vi "Emballage check code lu_FLATPROP.vi"(1 "tab pcs emballées historique":string[][](array[string])=[["112105740008090004", "01.01.2001 01:01:00", "55", "01234/08-01.01.01", "1", "0"], ["112105740008090006", "01.01.2001 01:01:00", "55", "56789/08-01.01.01", "3", "0"], ["112105740008090007", "01.01.2001 01:01:00", "55", "56789/08-01.01.01", "4", "0"], ["112105740008090007", "01.01.2001 01:01:00", "55", "00123/08-01.01.01", "2", "1"]], 2 "error in":errorcluster caption="entrée d'erreur", 3 "n° lot à scanner":string="0808", 4 "chaîne lue par le lecteur IN":string="112105740008090004", 5 "tab pcs déjà emballées (histo+actu)":string[](array[string])=["112105740008090009", "112105740008090004", "112105740008090006", "112105740008090007", "112105740008090007R1"], 6 "Quantité du lot de livraison":string="200", 11 "Pb réseau GPAO":bool, 16 "n° commande EC":string="R03838/08-01.01.01") -> (9 "error out":errorcluster caption="sortie d'erreur", 13 "offset sur code bar début index":i16=-1, 14 "largeur index":i16=-1, 15 "Date production de la piéce":string, 17 "chaîne lue par le lecteur OUT":string="112105740008090004R1", 18 "Arrêter la série (T)":bool, 19 "Paramètres OK(=> T)":bool)   [LabVIEW 2020]
uses:
  Instance           3 31Saved   Emballage check code lu .vi
  VG_VerifTests_ModeRetour.vi
  Modules/FS/60_FS_Controles/60_FS_SetGet.ctl
panel:
  out "Glissière 2":u8(slide)=100 caption="Identification terminé." scale=0.0..100.0
  out "RETOUR CLIENT":string="1"
  # "dans historique :\ncolonne 0 = numéro de pièce\ncolonne 1 = date\ncolonne 2 = visa emball\ncolonne 3 = No commande\ncolonne 4 = carton\ncolonne 5 = qtté cmdée ou RC"
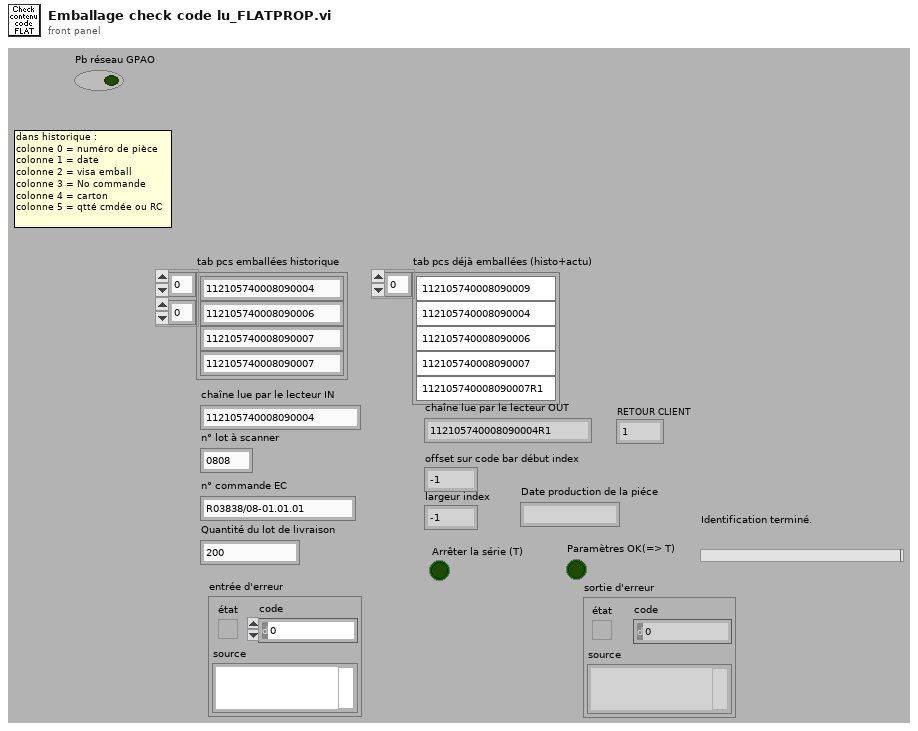
[diagram p1: front panel]
types:
  T1 = typedef "60_FS_SetGet.ctl" = enum16{"set", "get"}
  T2 = typedef "60_FS_CLT_Chemins.ctl" = cluster{"Racine_local":path, "Racine_reseau":path, "Racine_Support_Application":path, "Fichier_Journalisation":path, "Connexion_BDD_VSX":path, "Connexion_BDD_PLZ":path}
  T3 = typedef "Emballage_BDD_param_Produit.ctl" = cluster{"No_Valve_FAS":string, "suffixe":string, "designation":string, "indice_produit":string, "code_barre_fixe":string, "affiche_code_barre_client":string, "affiche_no_client":string, "Nb_vlve_par_carton":u16, "melange_des_lots_possible":string, "id_article":string, "Indice_Rev":string, "Famille":string, "date":string, "code_barre_fixe_Fin":string, "Longeur_No_Serie":string}
  T4 = typedef "DATA Valve.ctl" = cluster{"Existe ?":bool, "N° Valve":string, "Valve Codif":string, "Résultat test Hyst.":i32, "Résultat test Fuite":i32, "ID Valid Flatprop M":i32, "Date test Hyst.":string, "Date Test Fuite":string, "Date Emballage":string, "Historique Test Hyst.":string, "Historique Tes Fuite":string, "N° RETOUR":string, "Résultat test Dielec.":i32, "Date Test Dielec.":string, "R Test Dielec.[Ohm]":dbl, "Ifuite Test Dielec. [mA]":dbl, "Q Test Dielec.[L/mn]":dbl, "N°Valve sans Embase":string}
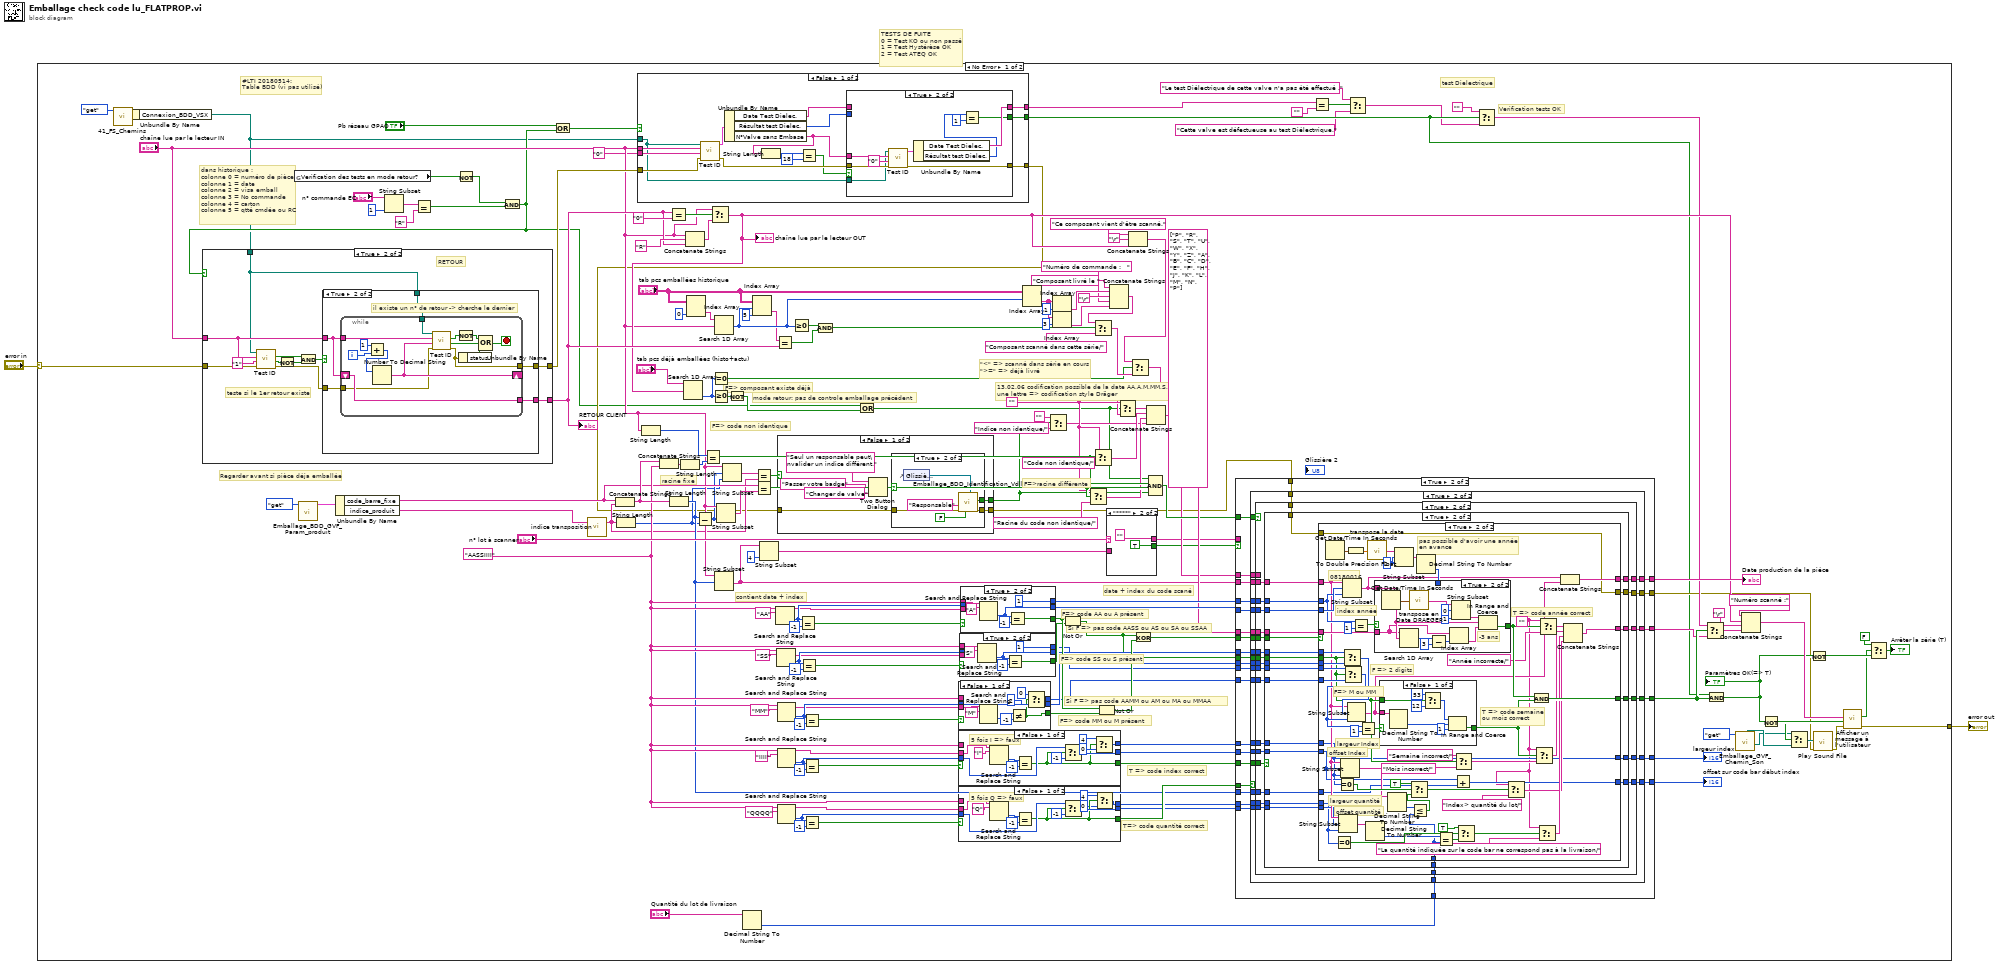
[diagram p0: block diagram]
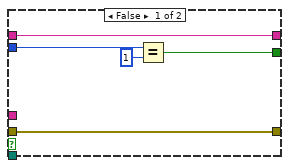
[diagram p2: hidden frame]
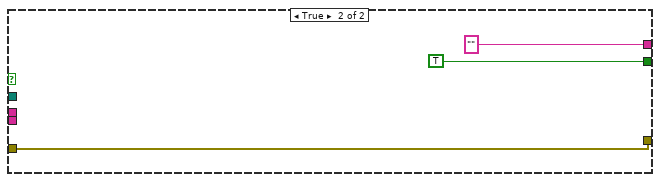
[diagram p3: hidden frame]
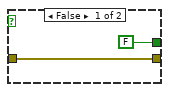
[diagram p4: hidden frame]
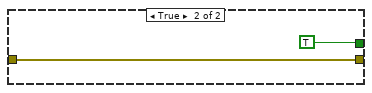
[diagram p5: hidden frame]
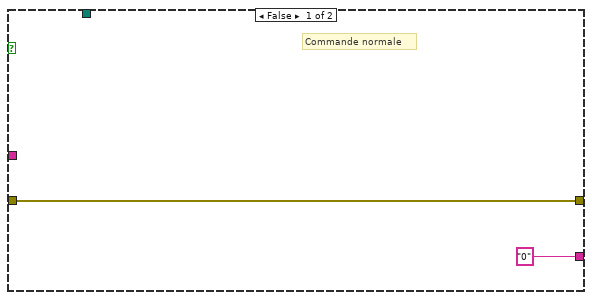
[diagram p6: hidden frame]
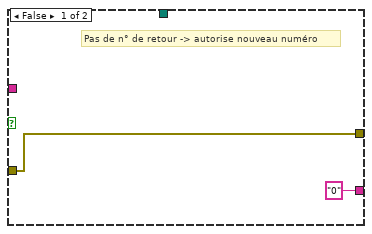
[diagram p7: hidden frame]
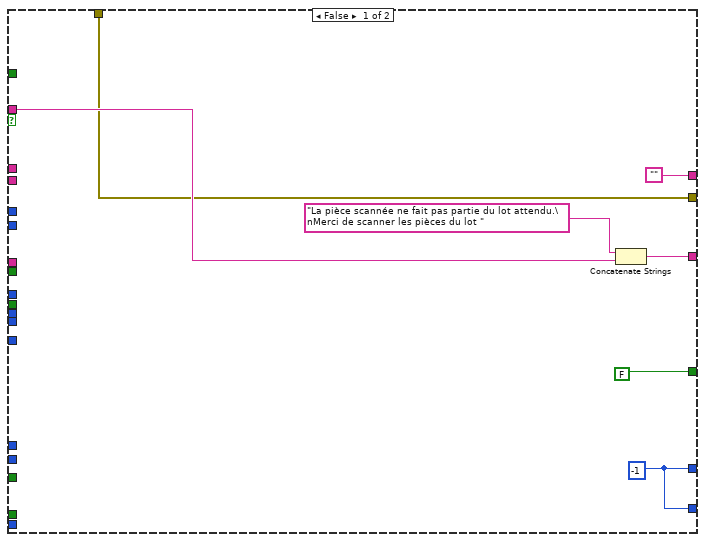
[diagram p8: hidden frame]
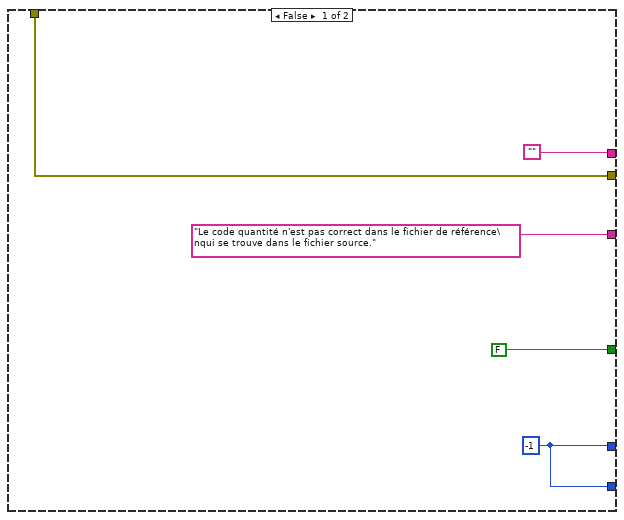
[diagram p9: hidden frame]
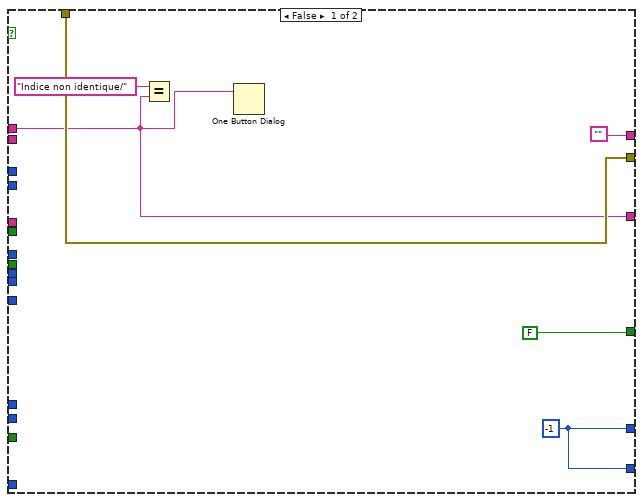
[diagram p10: hidden frame]
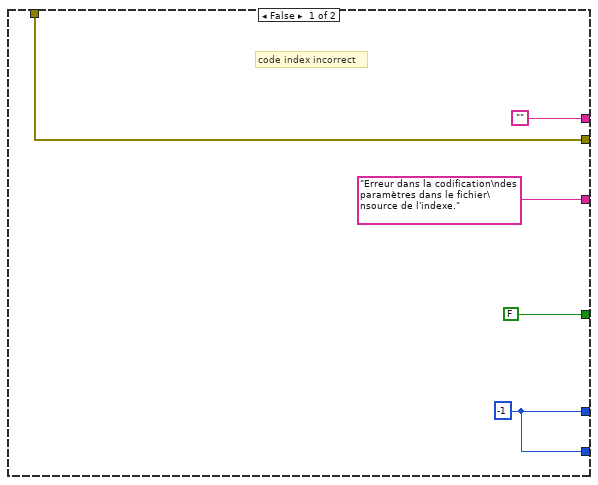
[diagram p11: hidden frame]
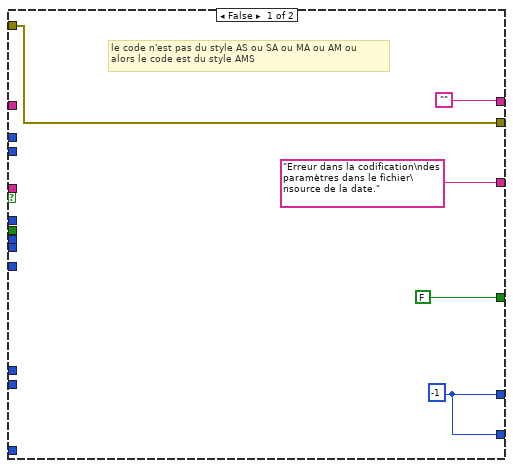
[diagram p12: hidden frame]
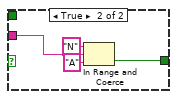
[diagram p13: hidden frame]
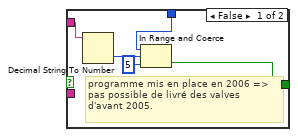
[diagram p14: hidden frame]
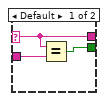
[diagram p15: hidden frame]
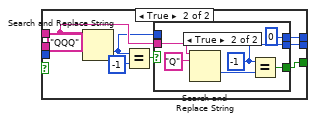
[diagram p16: hidden frame]
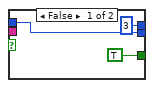
[diagram p17: hidden frame]
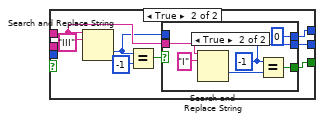
[diagram p18: hidden frame]
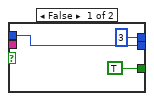
[diagram p19: hidden frame]
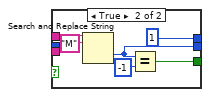
[diagram p20: hidden frame]
diagram:
  # "TESTS DE FUITE\n0 = Test KO ou non passé\n1 = Test Hystérèse OK\n2 = Test ATEQ OK"
  n1 = case shown="No Error" "error in" {
    selector: "error in" -> [w12 w577]
    tunnel: [w50 w577] -> w1
    frame No Error {
      w52 = "AASSIIII"
      w131 = ""
      # "#LTI 20180514:\nTable BDD (vi pas utilisé)"
      # "mode retour: pas de controle emballage précédent"
      # "Regarder avant si pièce déja emballée"
      # "Verification tests OK"
      # "test Dielectrique"
      # "dans historique :\ncolonne 0 = numéro de pièce\ncolonne 1 = date\ncolonne 2 = visa emball\ncolonne 3 = No commande\ncolonne 4 = carton\ncolonne 5 = qtté cmdée ou RC"
      # "\"<\" => scanné dans série en cours\n\">=\" => déjà livré"
      # "T=> code quantité correct"
      # "Si F => pas code AASS ou AS ou SA ou SSAA"
      # "Si F => pas code AAMM ou AM ou MA ou MMAA"
      # "F=> code MM ou M présent"
      # "F=> code SS ou S présent"
      # "F=> code AA ou A présent"
      # "T => code index correct"
      # "13.02.06 codification possible de la date AA,A,M,MM,S,SS\nune lettre => codification style Dräger"
      # "date + index du code scané"
      # "contient date + index"
      # "racine fixe"
      # "F=> composant existe déjà"
      # "F=> code non identique"
      # "F=>racine différente"
      n2 = call "41_FS_Chemins.vi"("SetGet"=60_FS_SetGet."get") -> ("CLT_Chemins_out"=w6:T2)  [unwired: 9 in, 1 out]
      n3 = Unbundle By Name(w6) -> ("Connexion_BDD_VSX"=w5:path)
      n4 = global read "VG_VerifTests_ModeRetour.vi" "Verification des tests en mode retour?"() -> (w14:bool)
      n5 = call "Emballage_BDD_GVF_Param_produit.vi"("Énum"=enum16{"set", "get"}."get") -> ("CLS_param_produit"=w3:T3)  [unwired: 7 in, 3 out]
      n6 = Unbundle By Name(w3) -> ("code_barre_fixe"=w42:string, "indice_produit"=w41:string)
      n7 = String Subset(string="n° commande EC", length (rest)=1 ("longueur (reste)")) -> (substring=w65:string)  [unwired: 1 in]
      n8 = Equal?(x=w65, y="R" ("expression régulière")) -> (x = y?=w23:bool)
      n9 = Not(x=w14) -> (.not. x?=w13:bool)
      n10 = And(x=w13, y=w23) -> (x .and. y?=w11:bool)
      n11 = case shown="True" w11 {
        tunnel: "chaîne lue par le lecteur IN" -> [_ w231]
        tunnel: ["0" ("expression régulière") w227] -> w54
        tunnel: w5 -> [_ w226]
        tunnel: w12 -> [w221 w225]
        tunnel: [w221 w223] -> w49
        frame False {
          # "Commande normale"
        }
        frame True {
          # "teste si le 1er retour existe"
          # "RETOUR"
          n12 = call "Test ID.vi"("error in"=w225, "NO_RETOUR"="1" ("expression régulière"), "NO_VALVE"=w231, "connection information"=w226) -> ("error out"=w224:errorcluster, "Erreur de\n comunication"=w229:bool, "Existe ?"=w233:bool)  [unwired: 1 out]
          n13 = Not(x=w229) -> (.not. x?=w228:bool)
          n14 = And(x=w233, y=w228) -> (x .and. y?=w232:bool)
          n15 = case shown="True" w232 {
            tunnel: w226 -> [_ w240]
            tunnel: w231 -> [_ w239]
            tunnel: ["0" ("expression régulière") w238] -> w227
            tunnel: w224 -> [w234 w237]
            tunnel: [w234 w236] -> w223
            frame False {
              # "Pas de n° de retour -> autorise nouveau numéro"
            }
            frame True {
              # "il existe un n° de retour -> cherche le dernier"
              n16 = while {
                tunnel: w239 -> [w247]
                shift-right: [w249] -> _
                shift-left: w239 -> [w248]
                tunnel: w240 -> [w251]
                tunnel: [w248] -> w238
                tunnel: w237 -> [w243]
                tunnel: [w242] -> w236
                i -> [w254]
                stop <- w246 stop-if-true
                n17 = Add(x=1, y=w254) -> (x+y=w252:i32)
                n18 = Number To Decimal String(number=w252) -> (decimal integer string=w249:string)  [unwired: 1 in]
                n19 = call "Test ID.vi"("error in"=w243, "NO_RETOUR"=w249, "NO_VALVE"=w247, "connection information"=w251) -> ("error out"=w242:errorcluster, "Erreur de\n comunication"=w253:bool, "Existe ?"=w245:bool)  [unwired: 1 out]
                n20 = Not(x=w245) -> (.not. x?=w244:bool)
                n21 = Unbundle By Name(w242) -> ("status"=w241:bool)
                n22 = Compound Arithmetic op=OR(w244, w253, w241) -> (w246:bool)
              }
            }
          }
        }
      }
      "RETOUR CLIENT" <- w54
      n23 = Or(x="Pb réseau GPAO", y=w11) -> (x .or. y?=w26:bool)
      n24 = call "indice transposition.vi"("indice entrée"=w41) -> ("indice corrigé"=w36:string)  [unwired: 1 in, 1 out]
      n25 = Concatenate Strings(w42, w36) -> (w80:string)
      n26 = String Length(string=w36) -> (length=w38:i32)
      n27 = case shown="False" w26 {
        tunnel: "chaîne lue par le lecteur IN" -> [w184 _]
        tunnel: "0" ("chaîne lue par le lecteur IN") -> [w183 _]
        tunnel: w5 -> [w175 _]
        tunnel: w49 -> [w182 w203]
        tunnel: [w180 w203] -> w29
        tunnel: [w173 "" ("Date Test Dielec.")] -> w22
        tunnel: [w172 TRUE] -> w19
        frame False {
          n28 = call "Test ID.vi"("error in"=w182, "NO_RETOUR"=w183, "NO_VALVE"=w184, "connection information"=w175) -> ("error out"=w181:errorcluster, "TEST ID VALID"=w185:T4)  [unwired: 2 out]
          n29 = Unbundle By Name(w185) -> ("Date Test Dielec."=w174:string, "Résultat test Dielec."=w171:i32, "N°Valve sans Embase"=w177:string)
          n30 = String Length(string=w177) -> (length=w179:i32)
          n31 = Equal?(x=w179, y=18) -> (x = y?=w176:bool)
          n32 = case shown="True" w176 {
            tunnel: w181 -> [w190 w199]
            tunnel: [w190 w198] -> w180
            tunnel: w177 -> [_ w196]
            tunnel: w175 -> [_ w195]
            tunnel: [w189 w194] -> w173
            tunnel: w174 -> [w189 _]
            tunnel: [w187 w191] -> w172
            tunnel: w171 -> [w186 _]
            frame False {
              n33 = Equal?(x=w186, y=1) -> (x = y?=w187:bool)
            }
            frame True {
              n34 = call "Test ID.vi"("error in"=w199, "NO_RETOUR"="0", "NO_VALVE"=w196, "connection information"=w195) -> ("error out"=w198:errorcluster, "TEST ID VALID"=w197:T4)  [unwired: 2 out]
              n35 = Unbundle By Name(w197) -> ("Date Test Dielec."=w194:string, "Résultat test Dielec."=w192:i32)
              n36 = Equal?(x=w192, y=1) -> (x = y?=w191:bool)
            }
          }
        }
        frame True {
        }
      }
      n37 = String Length(string="chaîne lue par le lecteur IN") -> (length=w169:i32)
      n38 = Concatenate Strings(w80, w52) -> (w170:string)
      n39 = Equal?(x=w54, y="0" ("chaîne")) -> (x = y?=w55:bool)
      n40 = String Length(string=w80) -> (length=w43:i32)
      n41 = String Length(string=w170) -> (length=w168:i32)
      n42 = Concatenate Strings("chaîne lue par le lecteur IN", "R" ("chaîne"), w54) -> (w53:string)
      n43 = Index Array(array="tab pcs emballées historique", index (col)=0) -> (element=w88:string[])  [unwired: 1 in]
      n44 = Subtract(x=w43, y=w38) -> (x-y=w39:i32)
      n45 = Equal?(x=w169, y=w168) -> (x = y?=w136:bool)
      n46 = Select(t="chaîne lue par le lecteur IN", s=w55, f=w53) -> (s? t:f=w51:string)
      "chaîne lue par le lecteur OUT" <- w51
      n47 = Search 1D Array(1D array="tab pcs déjà emballées (histo+actu)", element=w51) -> (index of element=w87:i32)  [unwired: 1 in]
      n48 = Equal To 0?(x=w87) -> (x = 0?=w84:bool)
      n49 = Greater Or Equal To 0?(x=w87) -> (x >= 0?=w135:bool)
      n50 = Search 1D Array(1D array=w88, element="chaîne lue par le lecteur IN") -> (index of element=w63:i32)  [unwired: 1 in]
      n51 = String Subset(string="chaîne lue par le lecteur IN", offset (0)=w43) -> (substring=w77:string)  [unwired: 1 in]
      n52 = String Subset(string="chaîne lue par le lecteur IN", length (rest)=w39) -> (substring=w167:string)  [unwired: 1 in]
      n53 = String Subset(string="chaîne lue par le lecteur IN", offset (0)=w39, length (rest)=w38) -> (substring=w37:string)
      n54 = Not(x=w135) -> (.not. x?=w134:bool)
      n55 = Decimal String To Number(string="Quantité du lot de livraison") -> (number=w122:i32)  [unwired: 2 in, 1 out]
      n56 = Index Array(array="tab pcs emballées historique", index (row)=w63, index (col)=5) -> (element=w61:string)
      n57 = Equal?(x=w42, y=w167) -> (x = y?=w137:bool)
      n58 = Equal?(x=w37, y=w36) -> (x = y?=w30:bool)
      n59 = String Subset(string=w77, length (rest)=4 ("longueur (reste)")) -> (substring=w72:string)  [unwired: 1 in]
      n60 = Equal?(x=w61, y=w54) -> (x = y?=w60:bool)
      n61 = Search and Replace String(input string=w52, search string="AA") -> (result string=w125:string, offset past replacement=w154:i32)  [unwired: 6 in, 2 out]
      n62 = Search and Replace String(input string=w52, search string="SS") -> (result string=w110:string, offset past replacement=w153:i32)  [unwired: 6 in, 2 out]
      n63 = case shown="False" w30 {
        tunnel: w29 -> [w210 w220]
        tunnel: [w209 w220] -> w28
        tunnel: [w208 TRUE] -> w27
        frame False {
          n64 = Two Button Dialog(message="Seul un responsable peut\nvalider un indice différent.", 1:"Changer de valve" ("Nom du bouton F (\"Annuler\")"), 2:"Passer votre badge" ("Nom du bouton V (\"OK\")")) -> (T button?=w207:bool)
          n65 = case shown="True" w207 {
            tunnel: w210 -> [w212 w215]
            tunnel: [w212 w214] -> w209
            tunnel: [FALSE ("OK") w213] -> w208
            frame False {
            }
            frame True {
              n66 = control-ref of="Glissière 2"() -> (w218:refnum<vi>)
              n67 = call "Emballage_BDD_Identification_Vdll.vi"("Glissière"=w218, "lecture seul possible ?"=FALSE, "error in"=w215, "Posage choisi"="Responsable" ("Posage choissi")) -> ("error Out"=w214:errorcluster, "OK"=w213:bool)  [unwired: 3 in, 3 out]
            }
          }
        }
        frame True {
        }
      }
      n68 = Search and Replace String(input string=w52, search string="MM") -> (result string=w109:string, offset past replacement=w152:i32)  [unwired: 6 in, 2 out]
      n69 = Search and Replace String(input string=w52, search string="IIII") -> (result string=w126:string, offset past replacement=w119:i32)  [unwired: 6 in, 2 out]
      n70 = Search and Replace String(input string=w52, search string="QQQQ") -> (result string=w117:string, offset past replacement=w116:i32)  [unwired: 6 in, 2 out]
      n71 = Greater Or Equal To 0?(x=w63) -> (x >= 0?=w59:bool)
      n72 = Equal?(x=w154, y=-1) -> (x = y?=w159:bool)
      n73 = Equal?(x=w153, y=-1) -> (x = y?=w160:bool)
      n74 = Equal?(x=w152, y=-1) -> (x = y?=w158:bool)
      n75 = Equal?(x=w119, y=-1) -> (x = y?=w155:bool)
      n76 = Equal?(x=w116, y=-1) -> (x = y?=w111:bool)
      n77 = And(x=w59, y=w60) -> (x .and. y?=w58:bool)
      n78 = Or(x=w11, y=w134) -> (x .or. y?=w24:bool)
      n79 = case shown="False" w155 {
        tunnel: w52 -> [_ w519]
        tunnel: [w505 w518] -> w120
        tunnel: w126 -> [w511 _]
        tunnel: w119 -> [w510 _]
        tunnel: [w508 w516] -> w118
        tunnel: [w504 w515] -> w113
        frame False {
          # "5 fois I => faux"
          n80 = Search and Replace String(input string=w511, search string="I") -> (offset past replacement=w512:i32)  [unwired: 6 in, 3 out]
          n81 = Equal?(x=w512, y=-1) -> (x = y?=w505:bool)
          n82 = Select(t=w510, s=w505, f=-1) -> (s? t:f=w508:i32)
          n83 = Select(t=4, s=w505, f=0) -> (s? t:f=w504:i32)
        }
        frame True {
          n84 = Search and Replace String(input string=w519, search string="III") -> (offset past replacement=w517:i32)  [unwired: 6 in, 3 out]
          n85 = Equal?(x=w517, y=-1) -> (x = y?=w520:bool)
          n86 = case shown="True" w520 {
            tunnel: w519 -> [_ w530]
            tunnel: [TRUE w528] -> w518
            tunnel: w517 -> [w524 _]
            tunnel: [w524 w527] -> w516
            tunnel: [3 0] -> w515
            frame False {
            }
            frame True {
              w527 = -1
              n87 = Search and Replace String(input string=w530, search string="I") -> (offset past replacement=w529:i32)  [unwired: 6 in, 3 out]
              n88 = Equal?(x=w527, y=w529) -> (x = y?=w528:bool)
            }
          }
        }
      }
      n89 = case shown="False" w111 {
        tunnel: w52 -> [_ w491]
        tunnel: [w479 w490] -> w115
        tunnel: w117 -> [w483 _]
        tunnel: w116 -> [w482 _]
        tunnel: [w480 w488] -> w114
        tunnel: [w476 w487] -> w112
        frame False {
          # "5 fois Q => faux"
          n90 = Search and Replace String(input string=w483, search string="Q") -> (offset past replacement=w484:i32)  [unwired: 6 in, 3 out]
          n91 = Equal?(x=w484, y=-1) -> (x = y?=w479:bool)
          n92 = Select(t=w482, s=w479, f=-1) -> (s? t:f=w480:i32)
          n93 = Select(t=4, s=w479, f=0) -> (s? t:f=w476:i32)
        }
        frame True {
          n94 = Search and Replace String(input string=w491, search string="QQQ") -> (offset past replacement=w489:i32)  [unwired: 6 in, 3 out]
          n95 = Equal?(x=w489, y=-1) -> (x = y?=w492:bool)
          n96 = case shown="True" w492 {
            tunnel: w491 -> [_ w502]
            tunnel: [TRUE w500] -> w490
            tunnel: w489 -> [w496 _]
            tunnel: [w496 w499] -> w488
            tunnel: [3 0] -> w487
            frame False {
            }
            frame True {
              w499 = -1
              n97 = Search and Replace String(input string=w502, search string="Q") -> (offset past replacement=w501:i32)  [unwired: 6 in, 3 out]
              n98 = Equal?(x=w499, y=w501) -> (x = y?=w500:bool)
            }
          }
        }
      }
      n99 = case shown="False" w158 {
        tunnel: w52 -> [_ w546]
        tunnel: [w533 w543] -> w151
        tunnel: [w540 w542] -> w143
        tunnel: w152 -> [w540 _]
        tunnel: [w535 1] -> w140
        tunnel: w109 -> [w536 _]
        frame False {
          n100 = Search and Replace String(input string=w536, search string="M") -> (offset past replacement=w539:i32)  [unwired: 6 in, 3 out]
          n101 = Not Equal?(x=w539, y=-1) -> (x != y?=w533:bool)
          n102 = Select(t=0, s=w533, f=2) -> (s? t:f=w535:i32)
        }
        frame True {
          n103 = Search and Replace String(input string=w546, search string="M") -> (offset past replacement=w542:i32)  [unwired: 6 in, 3 out]
          n104 = Equal?(x=w542, y=-1) -> (x = y?=w543:bool)
        }
      }
      n105 = case shown="True" w160 {
        tunnel: w52 -> [_ w561]
        tunnel: w153 -> [w555 _]
        tunnel: [w555 w558] -> w144
        tunnel: [w547 w557] -> w149
        tunnel: [w550 1] -> w141
        tunnel: w110 -> [w551 _]
        frame False {
          n106 = Search and Replace String(input string=w551, search string="S") -> (offset past replacement=w552:i32)  [unwired: 6 in, 3 out]
          n107 = Not Equal?(x=w552, y=-1) -> (x != y?=w547:bool)
          n108 = Select(t=0, s=w547, f=2) -> (s? t:f=w550:i32)
        }
        frame True {
          n109 = Search and Replace String(input string=w561, search string="S") -> (offset past replacement=w558:i32)  [unwired: 6 in, 3 out]
          n110 = Equal?(x=w558, y=-1) -> (x = y?=w557:bool)
        }
      }
      n111 = case shown="True" w159 {
        tunnel: w52 -> [_ w575]
        tunnel: w154 -> [w570 _]
        tunnel: [w570 w573] -> w146
        tunnel: [w562 w572] -> w150
        tunnel: [w565 1] -> w145
        tunnel: w125 -> [w568 _]
        frame False {
          n112 = Search and Replace String(input string=w568, search string="A") -> (offset past replacement=w566:i32)  [unwired: 6 in, 3 out]
          n113 = Not Equal?(x=w566, y=-1) -> (x != y?=w562:bool)
          n114 = Select(t=0, s=w562, f=2) -> (s? t:f=w565:i32)
        }
        frame True {
          n115 = Search and Replace String(input string=w575, search string="A") -> (offset past replacement=w573:i32)  [unwired: 6 in, 3 out]
          n116 = Equal?(x=w573, y=-1) -> (x = y?=w572:bool)
        }
      }
      n117 = Index Array(array="tab pcs emballées historique", index (row)=w63) -> (element=w90:string[])  [unwired: 1 in]
      n118 = Select(t="", s=w27, f="Indice non identique/") -> (s? t:f=w33:string)
      n119 = Index Array(array=w90, index=1) -> (element=w93:string)
      n120 = Index Array(array=w90, index=3) -> (element=w71:string)
      n121 = Not Or(1:w149, 2:w150) -> (0:w142:bool)
      n122 = Select(t=w131, s=w137, f="Racine du code non identique/") -> (s? t:f=w128:string)
      n123 = Select(t=w131, s=w136, f="Code non identique/") -> (s? t:f=w129:string)
      n124 = Not Or(1:w151, 2:w150) -> (0:w148:bool)
      n125 = case shown="\"****\"" "n° lot à scanner" {
        selector: "n° lot à scanner" -> [w471 _]
        tunnel: [w473 TRUE] -> w75
        tunnel: [w471 "" ("n° lot à scanner")] -> w74
        tunnel: w72 -> [w472 _]
        frame Default {
          n126 = Equal?(x=w471, y=w472) -> (x = y?=w473:bool)
        }
        frame "****" {
        }
      }
      n127 = Concatenate Strings("Composant livré le ", w93, "\r", "Numéro de commande :   ", w71) -> (w92:string)
      n128 = Select(t=w92, s=w58, f="Composant scanné dans cette série/") -> (s? t:f=w85:string)
      n129 = Concatenate Strings("Ce composant vient d'être scanné.", "\r", w51) -> (w82:string)
      n130 = Select(t=w82, s=w84, f=w85) -> (s? t:f=w86:string)
      n131 = Select(t=w131, s=w24, f=w86) -> (s? t:f=w130:string)
      n132 = Exclusive Or(1:w148, 2:w142) -> (0:w147:bool)
      n133 = Concatenate Strings(w130, w129, w128, w33) -> (w127:string)
      n134 = Compound Arithmetic op=AND(w24, w136, w137, w27) -> (w138:bool)
      n135 = case shown="True" w75 {
        tunnel: w147 -> [_ w288]
        tunnel: w146 -> [_ w287]
        tunnel: w145 -> [_ w286]
        tunnel: w144 -> [_ w285]
        tunnel: w143 -> [_ w284]
        tunnel: w142 -> [_ w283]
        tunnel: w141 -> [_ w282]
        tunnel: w140 -> [_ w281]
        tunnel: string[] ["P", "R", "S", "T", "U", "W", "X", "Y", "Z", "A", "B", "C", "D", "E", "F", "H", "J", "K", "L", "M", "N", "P"] -> [_ w280]
        tunnel: w138 -> [_ w279]
        tunnel: w127 -> [_ w278]
        tunnel: w122 -> [_ w277]
        tunnel: w120 -> [_ w276]
        tunnel: w118 -> [_ w275]
        tunnel: w115 -> [_ w274]
        tunnel: w114 -> [_ w273]
        tunnel: w113 -> [_ w272]
        tunnel: w112 -> [_ w271]
        tunnel: w43 -> [_ w270]
        tunnel: [w259 w269] -> w108
        tunnel: [w259 w268] -> w107
        tunnel: [w258 w267] -> w46
        tunnel: ["" w266] -> w98
        tunnel: [FALSE w265] -> w47
        tunnel: w77 -> [_ w264]
        tunnel: w74 -> [w256 _]
        tunnel: w28 -> [w255 w263]
        tunnel: [w255 w262] -> w32
        frame False {
          w259 = -1
          n136 = Concatenate Strings("La pièce scannée ne fait pas partie du lot attendu.\nMerci de scanner les pièces du lot ", w256) -> (w258:string)
        }
        frame True {
          n137 = case shown="True" w274 {
            tunnel: w276 -> [_ w319]
            tunnel: w288 -> [_ w318]
            tunnel: w287 -> [_ w317]
            tunnel: w286 -> [_ w316]
            tunnel: w285 -> [_ w315]
            tunnel: w284 -> [_ w314]
            tunnel: w283 -> [_ w313]
            tunnel: w282 -> [_ w312]
            tunnel: w281 -> [_ w311]
            tunnel: w264 -> [_ w310]
            tunnel: w280 -> [_ w309]
            tunnel: w279 -> [_ w308]
            tunnel: w278 -> [_ w307]
            tunnel: ["Le code quantité n'est pas correct dans le fichier de référence\nqui se trouve dans le fichier source." w306] -> w267
            tunnel: [FALSE w305] -> w265
            tunnel: w277 -> [_ w304]
            tunnel: w275 -> [_ w303]
            tunnel: w273 -> [_ w302]
            tunnel: w272 -> [_ w301]
            tunnel: w271 -> [_ w300]
            tunnel: ["" w299] -> w266
            tunnel: w270 -> [_ w298]
            tunnel: [w290 w297] -> w269
            tunnel: [w290 w296] -> w268
            tunnel: w263 -> [w289 w295]
            tunnel: [w289 w294] -> w262
            frame False {
              w290 = -1
            }
            frame True {
              n138 = case shown="True" w308 {
                tunnel: w319 -> [_ w349]
                tunnel: w318 -> [_ w348]
                tunnel: w317 -> [_ w347]
                tunnel: w316 -> [_ w346]
                tunnel: w315 -> [_ w345]
                tunnel: w314 -> [_ w344]
                tunnel: w313 -> [_ w343]
                tunnel: w312 -> [_ w342]
                tunnel: w311 -> [_ w341]
                tunnel: w310 -> [_ w340]
                tunnel: w309 -> [_ w339]
                tunnel: w307 -> [w320 _]
                tunnel: [w320 w337] -> w306
                tunnel: [FALSE w338] -> w305
                tunnel: w304 -> [_ w336]
                tunnel: w303 -> [_ w335]
                tunnel: w302 -> [_ w334]
                tunnel: w301 -> [_ w333]
                tunnel: w300 -> [_ w332]
                tunnel: ["" w331] -> w299
                tunnel: w298 -> [_ w330]
                tunnel: [w324 w329] -> w297
                tunnel: [w324 w328] -> w296
                tunnel: w295 -> [w322 w327]
                tunnel: [w322 w326] -> w294
                frame False {
                  w324 = -1
                  n139 = Equal?(x="Indice non identique/", y=w320) -> ()  [unwired: 1 out]
                  n140 = One Button Dialog(message=w320) -> ()  [unwired: 1 in, 1 out]
                }
                frame True {
                  n141 = case shown="True" w349 {
                    tunnel: w348 -> [_ w377]
                    tunnel: w347 -> [_ w376]
                    tunnel: w346 -> [_ w375]
                    tunnel: w345 -> [_ w374]
                    tunnel: w344 -> [_ w373]
                    tunnel: w343 -> [_ w372]
                    tunnel: w342 -> [_ w371]
                    tunnel: w341 -> [_ w370]
                    tunnel: w340 -> [_ w369]
                    tunnel: w339 -> [_ w368]
                    tunnel: [FALSE w367] -> w338
                    tunnel: ["Erreur dans la codification\ndes paramètres dans le fichier\nsource de l'indexe." w366] -> w337
                    tunnel: w336 -> [_ w365]
                    tunnel: w335 -> [_ w364]
                    tunnel: w334 -> [_ w363]
                    tunnel: w333 -> [_ w362]
                    tunnel: w332 -> [_ w361]
                    tunnel: ["" w360] -> w331
                    tunnel: w330 -> [_ w359]
                    tunnel: [w351 w358] -> w329
                    tunnel: [w351 w357] -> w328
                    tunnel: w327 -> [w350 w356]
                    tunnel: [w350 w355] -> w326
                    frame False {
                      w351 = -1
                      # "code index incorrect"
                    }
                    frame True {
                      n142 = case shown="True" w377 {
                        tunnel: w376 -> [_ w437]
                        tunnel: w375 -> [_ w429]
                        tunnel: w374 -> [_ w441]
                        tunnel: w373 -> [_ w440]
                        tunnel: w372 -> [_ w413]
                        tunnel: w371 -> [_ w439]
                        tunnel: w370 -> [_ w438]
                        tunnel: w369 -> [_ w409]
                        tunnel: w368 -> [_ w427]
                        tunnel: [FALSE w421] -> w367
                        tunnel: ["Erreur dans la codification\ndes paramètres dans le fichier\nsource de la date." w417] -> w366
                        tunnel: w365 -> [_ w396]
                        tunnel: w364 -> [_ w388]
                        tunnel: w363 -> [_ w408]
                        tunnel: w362 -> [_ w385]
                        tunnel: w361 -> [_ w407]
                        tunnel: ["" w389] -> w360
                        tunnel: w359 -> [_ w387]
                        tunnel: [w379 w386] -> w358
                        tunnel: [w379 w385] -> w357
                        tunnel: w356 -> [w378 w384]
                        tunnel: [w378 w384] -> w355
                        frame False {
                          w379 = -1
                          # "le code n'est pas du style AS ou SA ou MA ou AM ou\nalors le code est du style AMS"
                        }
                        frame True {
                          w383 = ""
                          w434 = 2
                          # "08180016"
                          # "largeur quantité"
                          # "largeur Index"
                          # "offset quantité"
                          # "offset Index"
                          # "T => code semaine\nou mois correct"
                          # "pas possible d'avoir une année\nen avance"
                          # "T => code année correct"
                          # "F=> M ou MM"
                          # "F => 2 digits"
                          # "index année"
                          n143 = Get Date/Time In Seconds() -> (seconds since 1Jan1904=w435:timestamp)
                          n144 = Equal To 0?(x=w407) -> (x = 0?=w406:bool)
                          n145 = Equal To 0?(x=w385) -> (x = 0?=w400:bool)
                          n146 = String Subset(string=w409, offset (0)=w408, length (rest)=w407) -> (substring=w402:string)
                          n147 = String Subset(string=w409, offset (0)=w388, length (rest)=w385) -> (substring=w398:string)
                          n148 = String Subset(string=w409, offset (0)=w437, length (rest)=w429) -> (substring=w391:string)
                          n149 = Select(t=w441, s=w413, f=w440) -> (s? t:f=w426:i32)
                          n150 = Select(t=w439, s=w413, f=w438) -> (s? t:f=w424:i32)
                          n151 = To Double Precision Float(number=w435) -> (double precision float=w436:dbl)
                          n152 = String Subset(string=w409, offset (0)=w426, length (rest)=w424) -> (substring=w390:string)
                          n153 = Equal?(x=w429, y=1) -> (x = y?=w428:bool)
                          n154 = Equal?(x=w424, y=1) -> (x = y?=w423:bool)
                          n155 = Decimal String To Number(string=w402) -> (number=w401:i32)  [unwired: 2 in, 1 out]
                          n156 = call "transpose la date.vi"("date a partir du 1 janvier 1904"=w436) -> ("Date:Semaine/année"=w433:string)
                          n157 = case shown="False" w423 {
                            tunnel: w390 -> [w449 w453]
                            tunnel: w413 -> [w445 _]
                            tunnel: [w442 w450] -> w419
                            frame False {
                              n158 = Decimal String To Number(string=w449) -> (number=w448:i32)  [unwired: 2 in, 1 out]
                              n159 = Select(t=53, s=w445, f=12) -> (s? t:f=w446:i32)
                              n160 = In Range and Coerce(upper limit=w446, x=w448, lower limit=1) -> (In Range?=w442:bool)  [unwired: 1 out]
                            }
                            frame True {
                              n161 = In Range and Coerce(upper limit="N", x=w453, lower limit="A") -> (In Range?=w450:bool)  [unwired: 1 out]
                            }
                          }
                          n162 = Decimal String To Number(string=w398) -> (number=w397:i32)  [unwired: 2 in, 1 out]
                          n163 = String Subset(string=w433, offset (0)=w434, length (rest)=w434) -> (substring=w432:string)
                          n164 = Less Or Equal?(x=w397, y=w396) -> (x <= y?=w395:bool)
                          n165 = Select(t=TRUE, s=w400, f=w395) -> (s? t:f=w394:bool)
                          n166 = Decimal String To Number(string=w432) -> (number=w431:i32)  [unwired: 2 in, 1 out]
                          n167 = case shown="True" w428 {
                            tunnel: w391 -> [w458 w465]
                            tunnel: w431 -> [w455 _]
                            tunnel: [w454 w466] -> w422
                            tunnel: w427 -> [_ w461]
                            frame False {
                              # "programme mis en place en 2006 =>\npas possible de livré des valves\nd'avant 2005."
                              n168 = Decimal String To Number(string=w458) -> (number=w457:i32)  [unwired: 2 in, 1 out]
                              n169 = In Range and Coerce(upper limit=w455, x=w457, lower limit=5) -> (In Range?=w454:bool)  [unwired: 1 out]
                            }
                            frame True {
                              # "-3 ans"
                              n170 = Get Date/Time In Seconds() -> (seconds since 1Jan1904=w459:timestamp)
                              n171 = Search 1D Array(1D array=w461, element=w465) -> (index of element=w464:i32)  [unwired: 1 in]
                              n172 = call "transpose en Date DRAEGER.vi"("horodatage"=w459) -> ("Date Dräger"=w468:string)
                              n173 = Subtract(x=w464, y=3) -> (x-y=w462:i32)
                              n174 = Index Array(array=w461, index=w462) -> (element=w460:string)
                              n175 = String Subset(string=w468, offset (0)=0, length (rest)=1) -> (substring=w467:string)
                              n176 = In Range and Coerce(upper limit=w467, x=w465, lower limit=w460) -> (In Range?=w466:bool)  [unwired: 1 out]
                            }
                          }
                          n177 = Equal?(x=w401, y=w396) -> (x = y?=w403:bool)
                          n178 = Add(x=w388, y=w387) -> (x+y=w386:i32)
                          n179 = Select(t="Semaine incorrect/", s=w413, f="Mois incorrect/") -> (s? t:f=w416:string)
                          n180 = Select(t=TRUE, s=w406, f=w403) -> (s? t:f=w405:bool)
                          n181 = Select(t=w383, s=w394, f="Index> quantité du lot/") -> (s? t:f=w392:string)
                          n182 = And(x=w422, y=w419) -> (x .and. y?=w421:bool)
                          n183 = Select(t=w383, s=w419, f=w416) -> (s? t:f=w418:string)
                          n184 = Select(t=w383, s=w405, f="La quantité indiquée sur le code bar ne correspond pas à la livraison/") -> (s? t:f=w410:string)
                          n185 = Select(t=w383, s=w422, f="Année incorrecte/") -> (s? t:f=w420:string)
                          n186 = Concatenate Strings(w391, w390) -> (w389:string)
                          n187 = Concatenate Strings(w420, w418, w410, w392) -> (w417:string)
                        }
                      }
                    }
                  }
                }
              }
            }
          }
        }
      }
      "Date production de la piéce" <- w98
      "offset sur code bar début index" <- w108
      "largeur index" <- w107
      n188 = Equal?(x=w22, y="") -> (x = y?=w21:bool)
      n189 = Select(t="Le test Diélectrique de cette valve n'a pas été effectué .", s=w21, f="Cette valve est défectueuse au test Diélectrrique.") -> (s? t:f=w15:string)
      n190 = Select(t="", s=w19, f=w15) -> (s? t:f=w44:string)
      n191 = Select(t=w44, s=w47, f=w46) -> (s? t:f=w45:string)
      n192 = And(x=w19, y=w47) -> (x .and. y?=w48:bool)
      "Paramètres OK(=> T)" <- w48
      n193 = call "Emballage_GVF_Chemin_Son.vi"("Énum"=enum16{"get", "set"}."get") -> ("Chemin lazer.WAV"=w9:path, "Chemin Utopia - Erreur.WAV"=w10:path)  [unwired: 6 in, 3 out]
      n194 = Concatenate Strings("Numéro scanné :", w51, "\r", w45) -> (w101:string)
      n195 = Not(x=w48) -> (.not. x?=w106:bool)
      n196 = Select(t=w9, s=w48, f=w10) -> (s? t:f=w79:path)
      n197 = Not(x=w48) -> (.not. x?=w105:bool)
      n198 = call <vilib>:"Play Sound File.vi"("error in (no error)"=w32, "path"=w79) -> ("error out"=w78:errorcluster)  [unwired: 8 in, 1 out]
      n199 = call "Afficher un message à l'utilisateur"("error in (no error)"=w78, "Enable"=w106, "Message"=w101) -> ("error out"=w50:errorcluster, "Continuer"=w102:bool)  [unwired: 7 in]
      n200 = Select(t=FALSE, s=w102, f=w105) -> (s? t:f=→"Arrêter la série (T)":bool)
    }
    frame Error {
    }
  }
  "error out" <- w1
